vi "My_Controls_Example_with_MathScript_VI.vi"() -> ()   [LabVIEW 2021]
uses:
  <vilib>/imath/engines/lvmath/Plug In/Control Design/BuiltInFunctions/tf/NIMS_CD_tf(num,den,Ts).vi
  <vilib>/imath/engines/lvmath/Plug In/Control Design/BuiltInFunctions/step/NIMS_CD_[Y,T]=step(TF,[Tinfo]).vi
  <vilib>/imath/engines/lvmath2/RunTimeEngine/NodeEndStatement/NIMS_NodeEndStatement_Get Vector.vi
  <instcachedir>/0/NIMS_NodeEndStatement_Get Vector_FBB85A4AFA7243FBA907ED20414130A8.lvgen/NIMS_NodeEndStatement_Get Vector_FBB85A4AFA7243FBA907ED20414130A8_001.vi
  <vilib>/imath/engines/lvmath2/RunTimeEngine/NodeEndStatement/NIMS_NodeEndStatement_Output.vi
  <instcachedir>/0/NIMS_NodeEndStatement_Output_53EC0D466D134D7ABD903AC30B43404B.lvgen/NIMS_NodeEndStatement_Output_53EC0D466D134D7ABD903AC30B43404B_005.vi
  <vilib>/imath/engines/lvmath2/RunTimeEngine/ErrorHandling/NIMS_Finalize Error.vi
panel:
  out "Waveform Graph":dbl[](graph)
  in  "stop":bool
  in  "Natural Frequency":dbl(slide) scale=0.0..5.0
  in  "Damping Ratio":dbl(slide) scale=0.0..1.0
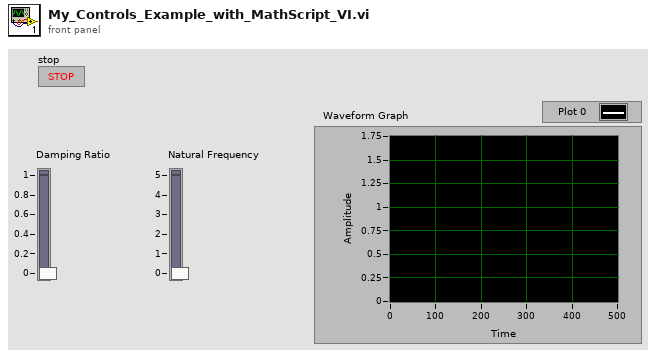
[diagram p1: front panel]
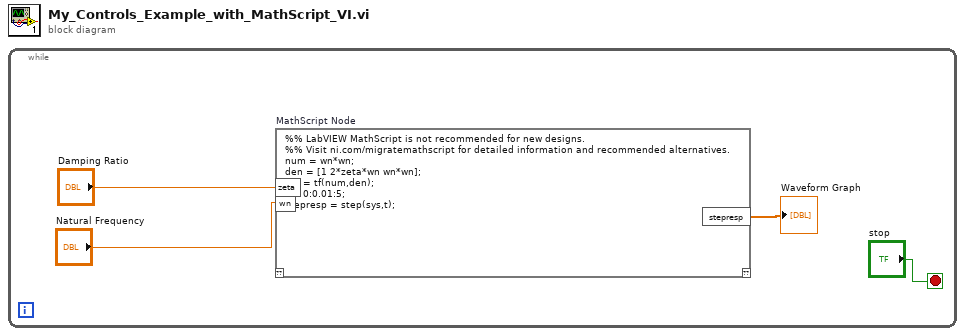
[diagram p0: block diagram]
diagram:
  n1 = while {
    stop <- "stop" stop-if-true
    n2 = mathscript code="%% LabVIEW MathScript is not recommended for new designs.\n%% Visit ni.com/migratemathscript for detailed information and recommended alternatives.\nnum = wn*wn;\nden = [1 2*zeta*wn wn*wn];\nsys = tf(num,den);\nt = 0:0.01:5;\nstepresp = step(sys,t);"("wn"="Natural Frequency", "zeta"="Damping Ratio") -> ("stepresp"=→"Waveform Graph":dbl[])  [unwired: 1 in, 1 out]
  }
